vi "contador.vi"(8 "Opciones":enum16{"reset", "mas uno", "lectura"}(ring)) -> (0 "Contador":i32)   [LabVIEW 2017]
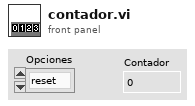
[diagram p1: front panel]
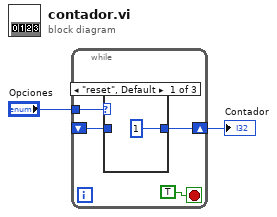
[diagram p0: block diagram]
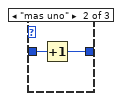
[diagram p2: hidden frame]
diagram:
  n1 = while {
    tunnel: "Opciones" -> [w6]
    shift-right: [w4] -> w1
    shift-left: _ -> [w3]
    stop <- TRUE stop-if-true
    n2 = case shown="\"reset\", Default" w6 {
      tunnel: [1 w8 w10] -> w4
      tunnel: w3 -> [_ w9 w10]
      frame "reset", Default {
      }
      frame "mas uno" {
        n3 = Increment(x=w9) -> (x+1=w8:i32)
      }
      frame "lectura" {
      }
    }
  }
  "Contador" <- w1
